vi "startSweepAndWait.vi"(8 "error in (no error)":errorcluster, 10 "time (s) [10 s]":dbl=10.0, 11 "Instrument.Lockin in":refnum<class "Instrument.Lockin.lvclass">) -> (0 "error out":errorcluster, 3 "Instrument.Lockin out":refnum<class "Instrument.Lockin.lvclass">)   [LabVIEW 2019, in "Instrument.Lockin.lvlib" / "Instrument.Lockin.lvclass"]
doc: "Starts a sweep and waits for it to be finished (up to <b>time</b>)"
uses:
  Instrument.Lockin.lvclass
  <userlib>/LevyLab/Instrument Framework/Instrument Types/Lockin/Instrument.LockinAPI.lvclass
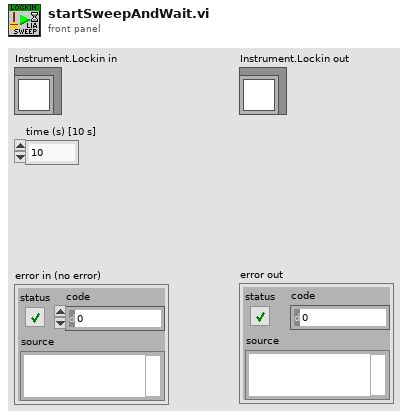
[diagram p1: front panel]
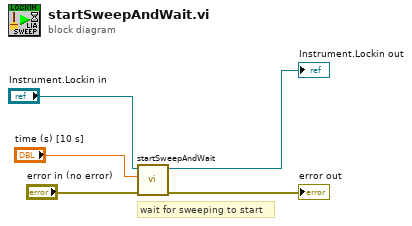
[diagram p0: block diagram]
diagram:
  # "wait for sweeping to start"
  n1 = call-parent "startSweepAndWait.vi"("error in (no error)"="error in (no error)", "time (s) [10 s]"="time (s) [10 s]", "Instrument.LockinAPI in"="Instrument.Lockin in") -> ("error out"=→"error out":errorcluster, "Instrument.LockinAPI out"=→"Instrument.Lockin out":refnum<class "Instrument.Lockin.lvclass">)  [unwired: 7 in]
